vi "Edit Sample Metadata.vi"(11 "Error In":errorcluster) -> (4 "MetaData File":path, 15 "Error Out":errorcluster)   [LabVIEW 2016]
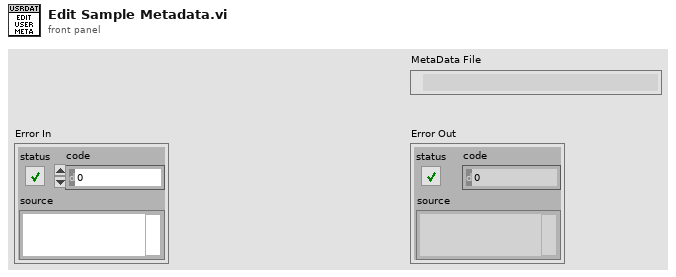
[diagram p1: front panel]
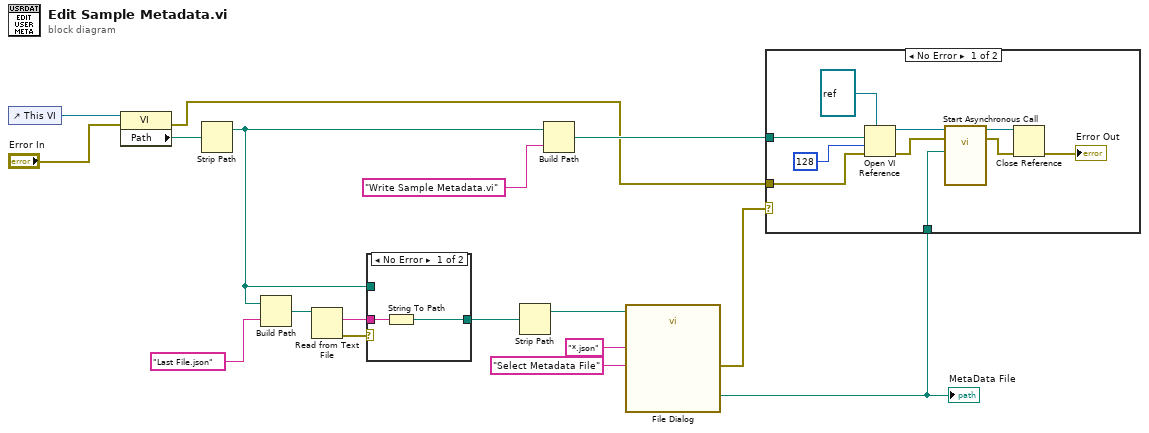
[diagram p0: block diagram]
diagram:
  n1 = control-ref of="This VI"() -> (w17:refnum<vi>)
  n2 = property class="VI"(reference=w17, error in="Error In") -> (error out=w12:errorcluster, "Path"=w16:path)  [unwired: 1 out]
  n3 = Strip Path(path=w16) -> (stripped path=w1:path)  [unwired: 1 out]
  n4 = Build Path(base path=w1, name or relative path="Last File.json") -> (appended path=w10:path)
  n5 = Read from Text File(file (use dialog)=w10) -> (text=w3:string, error out=w4:errorcluster)  [unwired: 3 in, 2 out]
  n6 = case shown="No Error" w4 {
    tunnel: w3 -> [w19 _]
    tunnel: [w18 w20] -> w2
    tunnel: w1 -> [_ w20]
    frame No Error {
      n7 = String To Path(string=w19) -> (path=w18:path)
    }
    frame Error {
    }
  }
  n8 = Strip Path(path=w2) -> (stripped path=w7:path)  [unwired: 1 out]
  n9 = Build Path(base path=w1, name or relative path="Write Sample Metadata.vi") -> (appended path=w14:path)
  n10 = call "File Dialog"("start path"=w7, "prompt"="Select Metadata File", "pattern label"="*.json") -> ("selected path"=w6:path, "error out"=w5:errorcluster)  [unwired: 9 in, 2 out]
  "MetaData File" <- w6
  n11 = case shown="No Error" w5 {
    tunnel: w14 -> [w30 _]
    tunnel: w12 -> [w22 _]
    tunnel: w6 -> [w21 _]
    frame No Error {
      n12 = Open VI Reference(type specifier VI Refnum (for type only)=refnum<vi> refnum, vi path=w30, options=128, error in (no error)=w22) -> (vi reference=w27:refnum<vi>, error out=w25:errorcluster)  [unwired: 2 in]
      n13 = call-by-ref "Start Asynchronous Call"(reference=w27, error in=w25, "File Path"=w21) -> (reference out=w26:refnum<vi>, error out=w24:errorcluster)  [unwired: 12 in, 3 out]
      n14 = Close Reference(reference=w26, error in (no error)=w24) -> (error out=→"Error Out":errorcluster)
    }
    frame Error {
    }
  }
